vi "TestExec.UUT, Dir.vi"(7 "Module Q Name":string, 8 "error in":errorcluster, 10 "UUT Dir":path, 11 "Q In":refnum<queue>) -> (0 "error out":errorcluster)   [LabVIEW 2018]
uses:
  <vilib>/KATE/Queues/Q.Element.ctl
  <vilib>/KATE/Queues/Queue Utils.lvlib
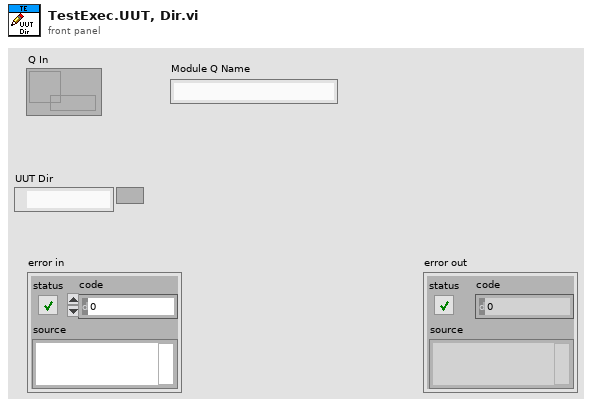
[diagram p1: front panel]
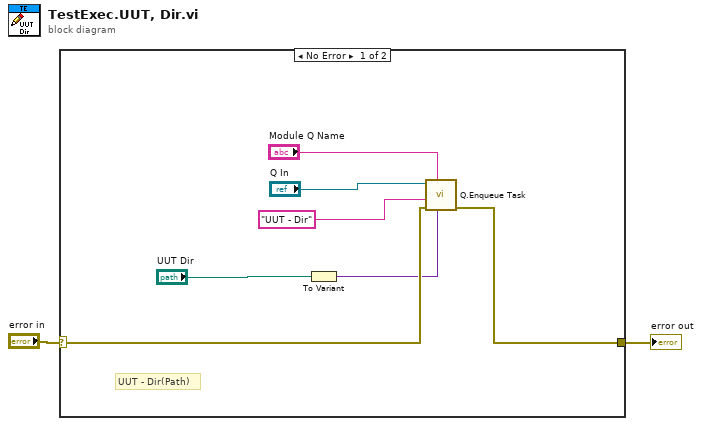
[diagram p0: block diagram]
diagram:
  n1 = case shown="No Error" "error in" {
    selector: "error in" -> [w6 w10]
    tunnel: [w7 w10] -> w1
    frame No Error {
      # "UUT - Dir(Path)"
      n2 = To Variant(anything="UUT Dir") -> (Variant=w5:variant)
      n3 = call <vilib>:"Q.Enqueue Task.vi"("Data1"=w5, "Q Name"="Module Q Name", "Error In"=w6, "Task Name"="UUT - Dir" ("Cmd"), "Q In"="Q In") -> ("error out"=w7:errorcluster)  [unwired: 5 in, 1 out]
    }
    frame Error {
    }
  }
  "error out" <- w1
